vi "vacuum_fgv.vi"(7 "cmd":enum16{"config", "start", "read", "close"}(ring), 8 "error in (no error)":errorcluster caption="에러 입력(에러 없음)") -> (0 "error out":errorcluster caption="에러 출력", 3 "data":waveform(dbl) caption="데이터")   [LabVIEW 2013]
uses:
  <vilib>/DAQmx/read.llb/DAQmx Read (Analog Wfm 1Chan NSamp).vi
  <vilib>/DAQmx/create/channels.llb/DAQmx Create Channel (AI-Voltage-Basic).vi
  <vilib>/DAQmx/configure/timing.llb/DAQmx Timing (Sample Clock).vi
  <vilib>/DAQmx/miscellaneous.llb/DAQmx Fill In Error Info.vi
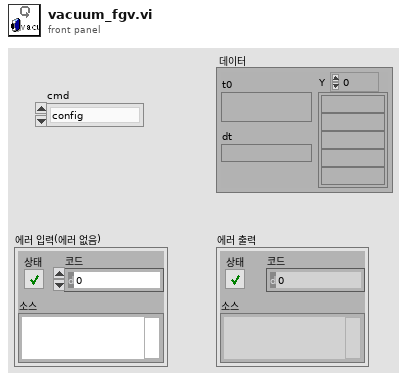
[diagram p1: front panel]
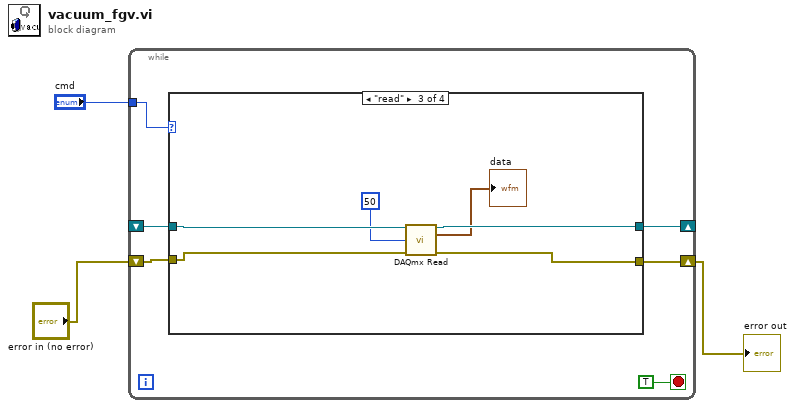
[diagram p0: block diagram]
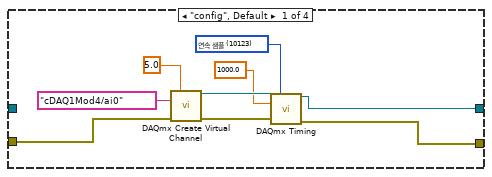
[diagram p2: hidden frame]
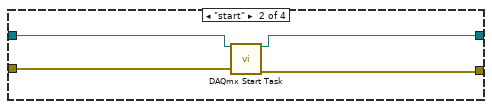
[diagram p3: hidden frame]
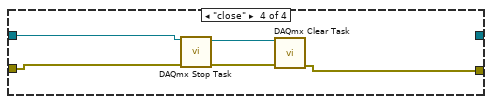
[diagram p4: hidden frame]
diagram:
  n1 = while {
    tunnel: "cmd" -> [w8]
    shift-right: [w6] -> w1
    shift-left: "error in (no error)" -> [w7]
    shift-right: [w5] -> _
    shift-left: _ -> [w4]
    stop <- TRUE stop-if-true
    n2 = case shown="\"read\"" w8 {
      tunnel: w7 -> [w18 w22 w27 w33]
      tunnel: [w15 w21 w28 w31] -> w6
      tunnel: [w13 w20 w25 _] -> w5
      tunnel: w4 -> [_ w19 w26 w29]
      frame "config", Default {
        w12 = 10123 items=["유한 샘플"=10178, "연속 샘플"=10123, "하드웨어 타이밍에 의한 단일 포인트"=12522] ("sample mode")
        n3 = call-poly <vilib>:"DAQmx Create Virtual Channel.vi"("maximum value"=5.0, "physical channels"=tag "cDAQ1Mod4/ai0", "error in"=w18) -> ("task out"=w14:refnum<k21>, "error out"=w16:errorcluster)  [unwired: 11 in]
        n4 = call-poly <vilib>:"DAQmx Timing.vi"("task/channels in"=w14, "sample mode"=w12, "rate"=1000.0, "error in"=w16) -> ("task out"=w13:refnum<k21>, "error out"=w15:errorcluster)  [unwired: 10 in]
      }
      frame "start" {
        n5 = call <vilib>:"DAQmx Start Task.vi"("task/channels in"=w19, "error in"=w22) -> ("task out"=w20:refnum<k21>, "error out"=w21:errorcluster)  [unwired: 12 in]
      }
      frame "read" {
        n6 = call-poly <vilib>:"DAQmx Read.vi"("task/channels in"=w26, "number of samples per channel"=50, "error in"=w27) -> ("task out"=w25:refnum<k21>, "data"=→"data":waveform(dbl), "error out"=w28:errorcluster)  [unwired: 10 in]
      }
      frame "close" {
        n7 = call <vilib>:"DAQmx Stop Task.vi"("task/channels in"=w29, "error in"=w33) -> ("task out"=w30:refnum<k21>, "error out"=w32:errorcluster)  [unwired: 12 in]
        n8 = call <vilib>:"DAQmx Clear Task.vi"("task in"=w30, "error in"=w32) -> ("error out"=w31:errorcluster)  [unwired: 13 in]
      }
    }
  }
  "error out" <- w1
